vi "OldByHang.vi"() -> ()   [LabVIEW 2022 SP3]
uses:
  <vilib>/Analysis/3filter.llb/Filter Passband Type.ctl
  <vilib>/Instr/_visa.llb/VISA Configure Serial Port (Instr).vi
  <vilib>/Analysis/3filter.llb/Butterworth Filter (DBL).vi
  <vilib>/measure/madcrms.llb/Basic Averaged DC-RMS for 1 Chan.vi
  <vilib>/Utility/file.llb/Read Delimited Spreadsheet (DBL).vi
  <vilib>/measure/maspectr.llb/FFT Power Spectrum and PSD for 1 Chan.vi
  <vilib>/Analysis/NI_AALBase.lvlib
  <vilib>/measure/NI_MAPro.lvlib
  <vilib>/measure/NI_MABase.lvlib
panel:
  in  "file path (dialog if empty)":path=path "D:/test.txt"
  out "数值 4":dbl
  in  "数值 3":dbl
  out "数值":dbl
  out "波形图":waveform(dbl)(graph)
  out "Power Spectrum / PSD":cluster{"f0":dbl, "df":dbl, "magnitude":dbl[]} caption="功率谱/PSD" {"magnitude" format="%.2p"; "f0" format="%0.2p"; "df" format="%0.2p"}
  out "回放2":dbl[](graph)
  out "波形图 3":dbl[](graph)
  out "错误输出":errorcluster
  in  "VISA resource name":refnum<visa-resource-name>="COM7" caption="VISA资源名称"
  out "读取缓冲区":string
  out "*(类型 *) &x":u16
  out "波形图表":i32(graph)
  in  "停止":bool
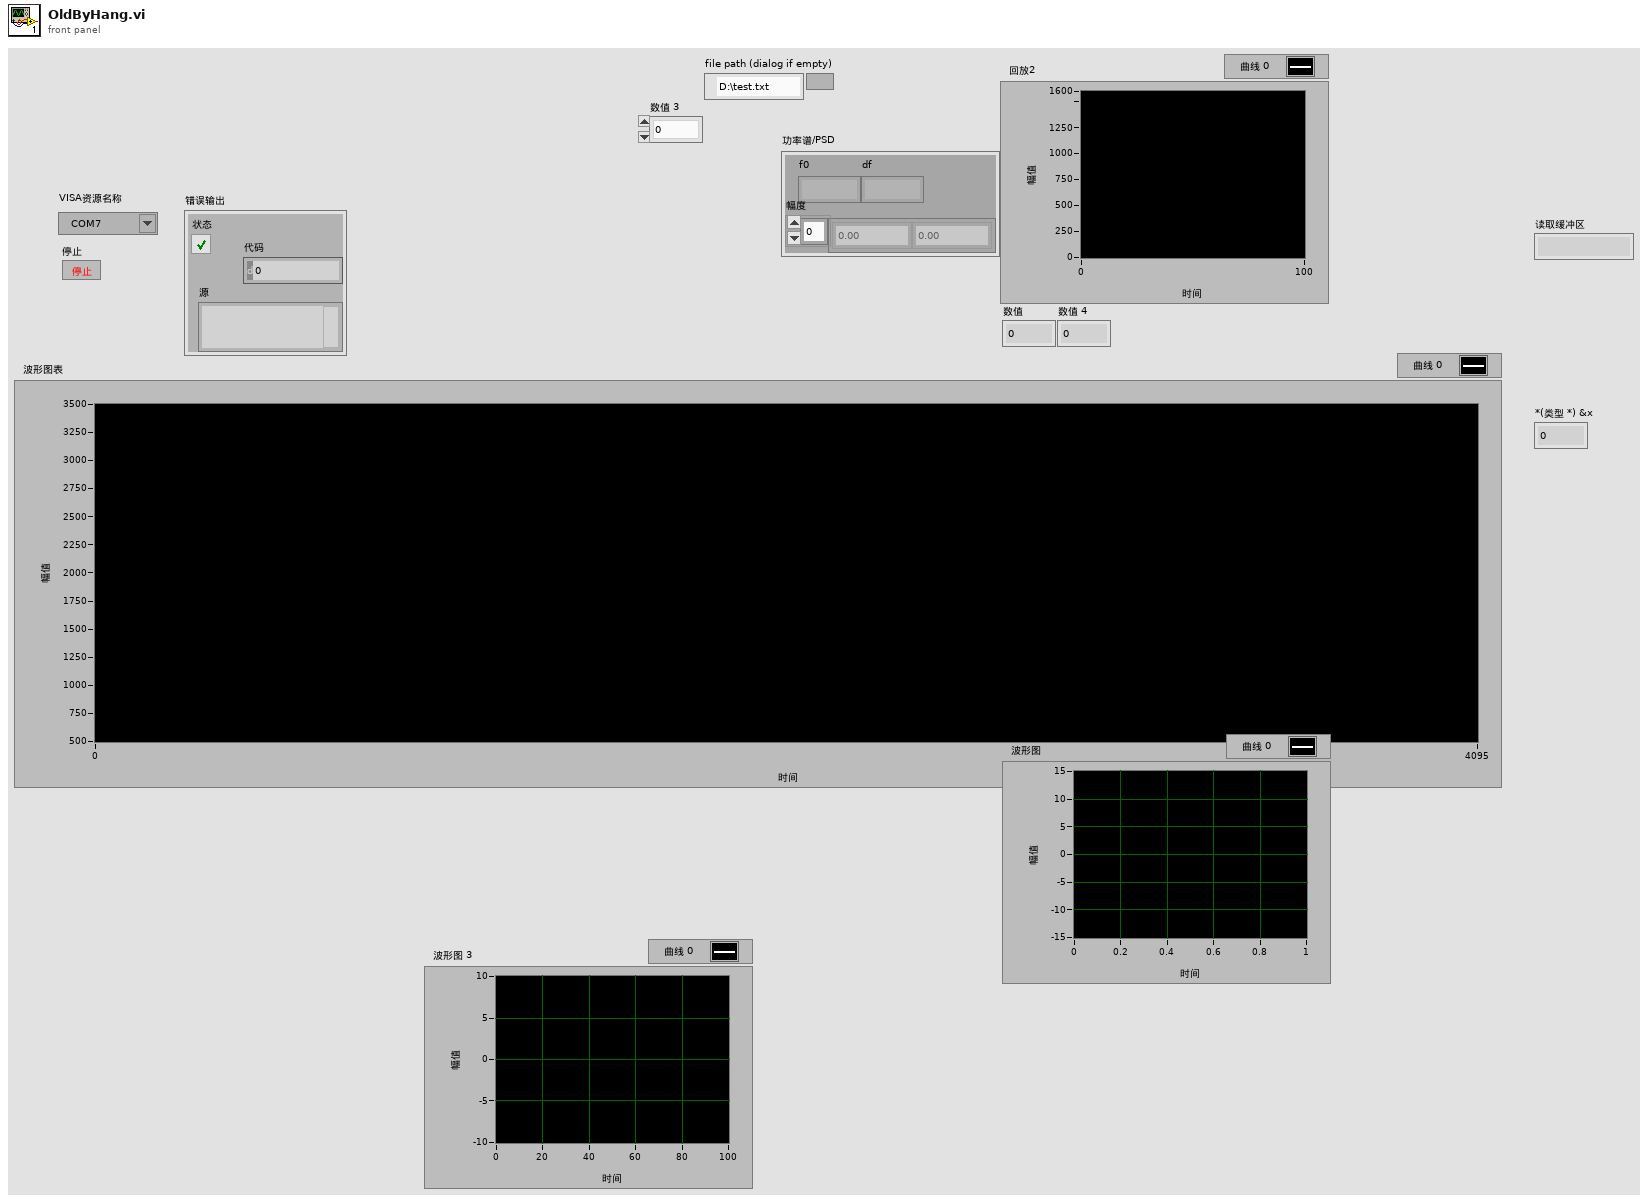
[diagram p1: front panel]
types:
  T1 = typedef "NI_AALBase.lvlib/Filter Passband Type.ctl" = enum32{"Lowpass", "Highpass", "Bandpass", "Bandstop"}
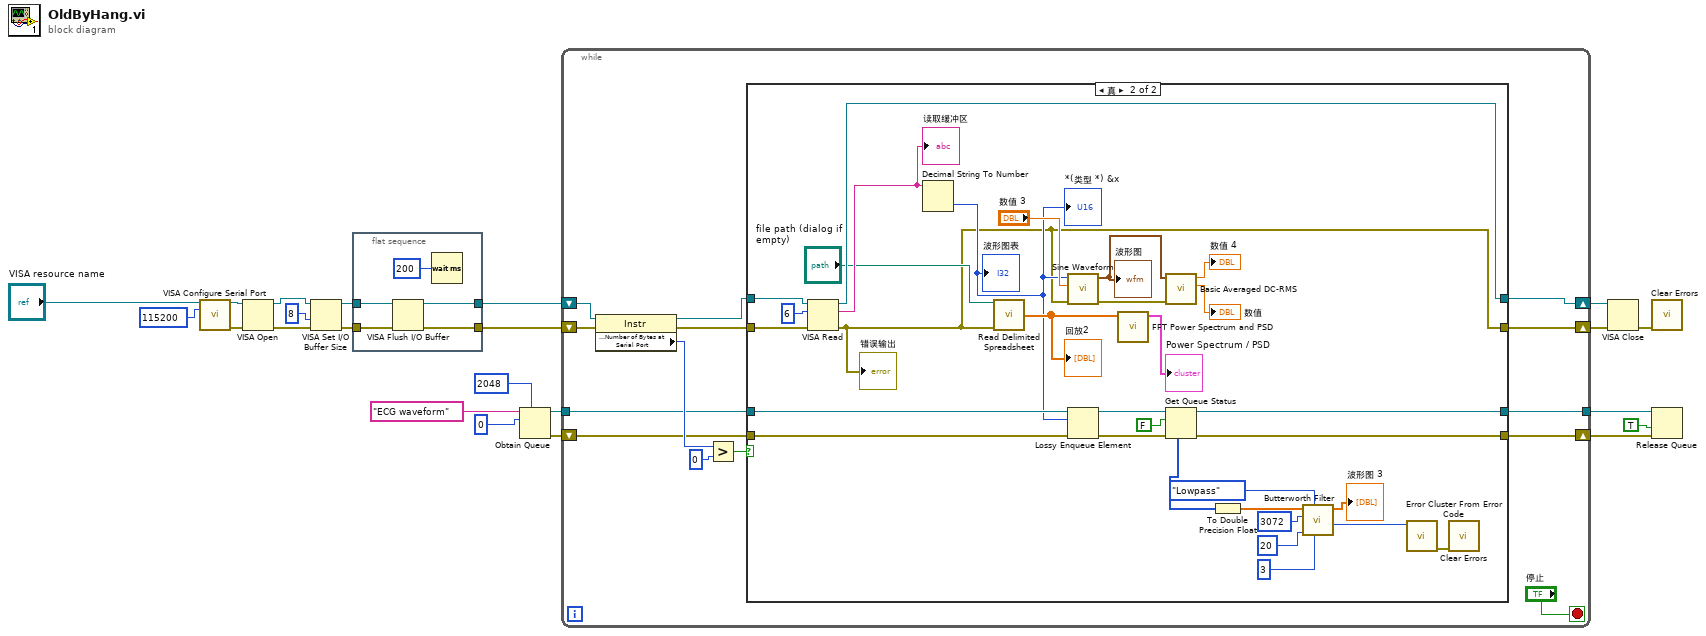
[diagram p0: block diagram]
diagram:
  n1 = call-poly "VISA Configure Serial Port"("VISA resource name"="VISA resource name", "baud rate (9600)"=u32 115200) -> ("VISA resource name out"=w16:refnum<visa-resource-name>, "error out"=w17:errorcluster)  [unwired: 12 in]
  n2 = VISA Open(error in (no error)=w17, VISA resource name=w16) -> (VISA resource name=w20:refnum<visa-resource-name>, error out=w19:errorcluster)  [unwired: 3 in]
  n3 = VISA Set I/O Buffer Size(VISA resource name=w20, size (4096)=u32 8 ("大小(4096)"), error in (no error)=w19) -> (VISA resource name out=w14:refnum<visa-resource-name>, error out=w15:errorcluster)  [unwired: 1 in]
  n4 = flat-sequence {
    tunnel: w14 -> [w26]
    tunnel: w15 -> [w25]
    tunnel: [w24] -> w10
    tunnel: [w23] -> w9
    frame #0 {
      n5 = VISA Flush I/O Buffer(VISA resource name=w26, error in (no error)=w25) -> (VISA resource name out=w24:refnum<visa-resource-name>, error out=w23:errorcluster)  [unwired: 1 in]
      n6 = Wait (ms)(milliseconds to wait=u32 200 ("等待时间（毫秒）")) -> ()  [unwired: 1 out]
    }
  }
  n7 = Obtain Queue(max queue size (-1, unlimited)=2048 ("队列最大值（-1，无限）"), name (unnamed)="ECG waveform" ("名称（未命名）"), element data type=0) -> (queue out=w4:refnum<queue>, error out=w5:errorcluster)  [unwired: 2 in, 1 out]
  n8 = while {
    shift-right: [w41] -> w13
    shift-left: w10 -> [w38]
    shift-right: [w39] -> w12
    shift-left: w9 -> [w37]
    shift-right: [w28] -> w1
    shift-left: w5 -> [w30]
    tunnel: w4 -> [w31]
    tunnel: [w29] -> w2
    stop <- "停止" stop-if-true
    n9 = property class="Instr"(reference=w38, error in=w37) -> (reference out=w33:refnum<visa-resource-name>, error out=w34:errorcluster, "Serial Settings:Number of Bytes at Serial Port"=w36:u32)
    n10 = Greater?(x=w36, y=u32 0) -> (0:w32:bool)
    n11 = case shown="真" w32 {
      tunnel: [w44 w72] -> w41
      tunnel: [w45 w46] -> w39
      tunnel: w34 -> [w45 w74]
      tunnel: w33 -> [w44 w73]
      tunnel: w31 -> [w43 w61]
      tunnel: w30 -> [w42 w60]
      tunnel: [w43 w59] -> w29
      tunnel: [w42 w58] -> w28
      frame False {
      }
      frame True {
        n12 = VISA Read(VISA resource name=w73, byte count=u32 6 ("字节总数"), error in (no error)=w74) -> (VISA resource name out=w72:refnum<visa-resource-name>, read buffer=w75:string, error out=w46:errorcluster)  [unwired: 1 out]
        "读取缓冲区" <- w75
        "错误输出" <- w46
        n13 = Decimal String To Number(string=w75) -> (number=w47:i32)  [unwired: 2 in, 1 out]
        "*(类型 *) &x" <- w47
        "波形图表" <- w47
        n14 = call-poly <vilib>:"Read Delimited Spreadsheet.vi"("file path (dialog if empty)"="file path (dialog if empty)", "error in (no error)"=w46) -> ("first row"=w53:dbl[])  [unwired: 8 in, 5 out]
        "回放2" <- w53
        n15 = call <vilib>:"Sine Waveform.vi"("error in (no error)"=w46, "amplitude"="数值 3", "frequency"=w47) -> ("error out"=w52:errorcluster, "signal out"=w48:waveform(dbl))  [unwired: 7 in]
        "波形图" <- w48
        n16 = Lossy Enqueue Element(queue=w61, element=w47, error in (no error)=w60) -> (queue out=w63:refnum<queue>, error out=w64:errorcluster)  [unwired: 2 out]
        n17 = call-poly <vilib>:"FFT Power Spectrum and PSD.vi"("time signal"=w53) -> ("Power Spectrum / PSD"=→"Power Spectrum / PSD":cluster{"f0":dbl, "df":dbl, "magnitude":dbl[]})  [unwired: 7 in, 3 out]
        n18 = call-poly <vilib>:"Basic Averaged DC-RMS.vi"("error in (no error)"=w52, "signal in"=w48) -> ("RMS value"=→"数值":dbl, "DC value"=→"数值 4":dbl)  [unwired: 6 in, 2 out]
        n19 = Get Queue Status(queue=w63, return elements? (F)=FALSE, error in (no error)=w64) -> (queue out=w59:refnum<queue>, error out=w58:errorcluster, elements=w57:i32[])  [unwired: 5 out]
        n20 = To Double Precision Float(number=w57) -> (double precision float=w56:dbl[])
        n21 = call-poly <vilib>:"Butterworth Filter.vi"("order"=3, "filter type"=Filter_Passband_Type."Lowpass", "low cutoff freq: fl"=20, "sampling freq: fs"=3072, "X"=w56) -> ("error"=w67:i32, "Filtered X"=→"波形图 3":dbl[])  [unwired: 3 in]
        n22 = call <vilib>:"Error Cluster From Error Code.vi"("error code (0)"=w67) -> ("error out"=w71:errorcluster)  [unwired: 8 in]
        n23 = call <vilib>:"Clear Errors.vi"("error in (no error)"=w71) -> ()  [unwired: 5 in, 2 out]
      }
    }
  }
  n24 = VISA Close(VISA resource name=w13, error in (no error)=w12) -> (error out=w11:errorcluster)
  n25 = call <vilib>:"Clear Errors.vi"("error in (no error)"=w11) -> ()  [unwired: 5 in, 2 out]
  n26 = Release Queue(queue=w2, force destroy? (F)=TRUE, error in (no error)=w1) -> ()  [unwired: 3 out]
